vi "Python.vi"() -> ()   [LabVIEW 2024]
panel:
  in  "C":dbl format="%#_13g"
  out "F":dbl
  in  "error in (no error)":errorcluster
  out "error out":errorcluster
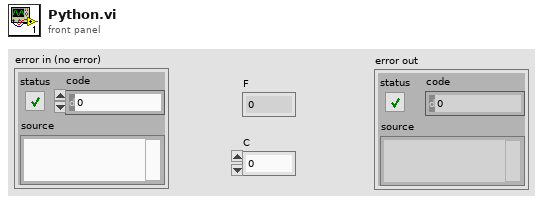
[diagram p1: front panel]
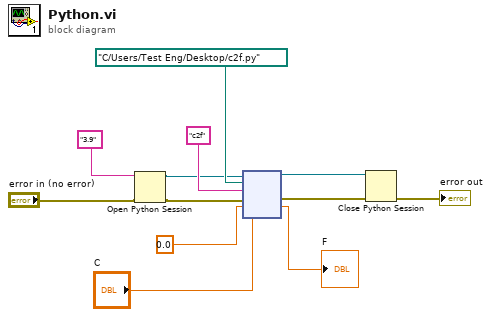
[diagram p0: block diagram]
diagram:
  n1 = Open Python Session(python version="3.9" ("Python version"), 3:"error in (no error)") -> (session out=w2:refnum<k35>, error out=w3:errorcluster)  [unwired: 1 in]
  n2 = node(w2, path "C:/Users/Test Eng/Desktop/c2f.py" ("module path"), "c2f" ("function name"), w3, 0.0, "C") -> (w11:refnum<k35>, w12:errorcluster, →"F":dbl)  [unwired: 1 in, 2 out]
  n3 = Close Python Session(session in=w11, error in=w12) -> (11:→"error out":errorcluster)
